vi "Create.vi"(8 "Error In":errorcluster) -> (0 "Error Out":errorcluster, 3 "Screen Out":refnum<class "Display.lvclass">)   [LabVIEW 2019, in "Display.lvclass"]
uses:
  Display.lvclass
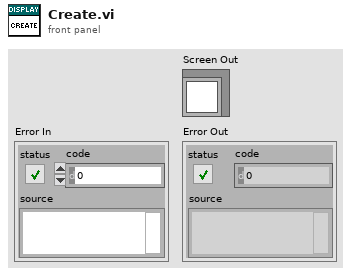
[diagram p1: front panel]
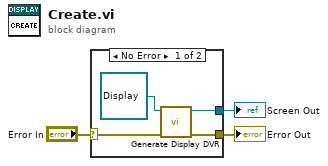
[diagram p0: block diagram]
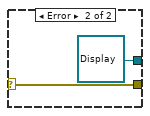
[diagram p2: hidden frame]
diagram:
  n1 = case shown="No Error" "Error In" {
    selector: "Error In" -> [w6 w9]
    tunnel: [w4 refnum<class "Display.lvclass"> refnum ("Screen.lvclass")] -> w3
    tunnel: [w5 w9] -> w1
    frame No Error {
      n2 = call "Generate Display DVR.vi"("Error In"=w6, "Display In"=refnum<class "Display.lvclass"> refnum ("Screen.lvclass")) -> ("Error Out"=w5:errorcluster, "Display Out"=w4:refnum<class "Display.lvclass">)  [unwired: 8 in]
    }
    frame Error {
    }
  }
  "Screen Out" <- w3
  "Error Out" <- w1
